vi "onStop.vi"(8 "error in (no error)":errorcluster, 11 "Client in":refnum<class "Client.lvclass">) -> (0 "error out":errorcluster, 3 "Client out":refnum<class "Client.lvclass">)   [LabVIEW 2013, in "MQTT Client.lvlib" / "Client.lvclass"]
uses:
  Client.lvclass
  Client.lvclass/Client.ctl
  MQTT_Base/Base Class/MQTT_Base.lvclass
  <vilib>/LabVIEW Open Source Project/MQTT Control Packets/Control Packets/PUBLISH/PUBLISH.lvclass
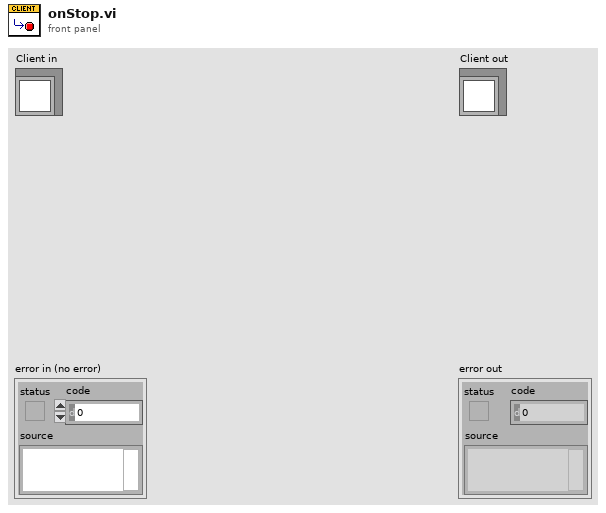
[diagram p1: front panel]
types:
  T1 = typedef "MQTT Client.lvlib/Client.lvclass/Public Events -- cluster.ctl" = cluster{"Connection Status":refnum<user-event>, "Connected":refnum<user-event>, "Application Message":refnum<user-event>}
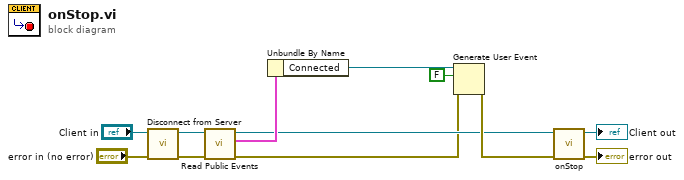
[diagram p0: block diagram]
diagram:
  n1 = call "Disconnect from Server.vi"("error in (no error)"="error in (no error)", "Client in"="Client in") -> ("error out"=w2:errorcluster, "Client out"=w4:refnum<class "Client.lvclass">)  [unwired: 7 in, 1 out]
  n2 = call "Read Public Events.vi"("error in (no error)"=w2, "Client in"=w4) -> ("error out"=w1:errorcluster, "Client Public Events"=w5:T1, "Client out"=w3:refnum<class "Client.lvclass">)  [unwired: 7 in]
  n3 = Unbundle By Name(w5) -> ("Connected"=w8:refnum<user-event>)
  n4 = Generate User Event(user event=w8, event data cluster=FALSE ("event data"), error in=w1) -> (error out=w7:errorcluster)  [unwired: 1 in, 1 out]
  n5 = call-parent "onStop.vi"("error in (no error)"=w7, "MQTT_Base in"=w3) -> ("error out"=→"error out":errorcluster, "MQTT_Base out"=→"Client out":refnum<class "Client.lvclass">)  [unwired: 8 in]
